vi "Acquisizione corse trigger.vi"() -> ()   [LabVIEW 2017]
uses:
  <vilib>/DAQmx/read.llb/DAQmx Read (Analog 1D Wfm NChan NSamp).vi
  <vilib>/Waveform/WDTOps.llb/WDT Index Channel DBL.vi
  <vilib>/Waveform/WDTOps.llb/WDT Append Waveforms DBL.vi
  <resource>/objmgr/daqmx.rc
  <vilib>/DAQmx/configure/timing.llb/DAQmx Timing (Sample Clock).vi
  <vilib>/DAQmx/configure/trigger.llb/DAQmx Start Trigger (Analog Edge).vi
  <vilib>/DAQmx/configure/trigger.llb/DAQmx Reference Trigger (Analog Edge).vi
panel:
  in  "source":string
  in  "rate":dbl=1000.0 format="%0.2f"
  in  "sample mode":i32(ring)=10178 items=["Finite Samples"=10178, "Continuous Samples"=10123, "Hardware Timed Single Point"=12522]
  in  "samples per channel":i32=1000
  in  "Save":bool
  out "error out":errorcluster
  in  "error in (no error)":errorcluster
  in  "valore di controllo 2":dbl=4.0
  in  "index 2":i32=2
  in  "valore di controllo":dbl=4.0
  in  "index":i32=2
  out "Photocell B":waveform(dbl)(graph)
  out "Photocell A":waveform(dbl)(graph)
  in  "Massa":string="_"
  out "photocell A":bool
  out "photocell B":bool
  in  "directory":path
  out "Load_Cell":waveform(dbl)(graph)
  in  "On/off":bool
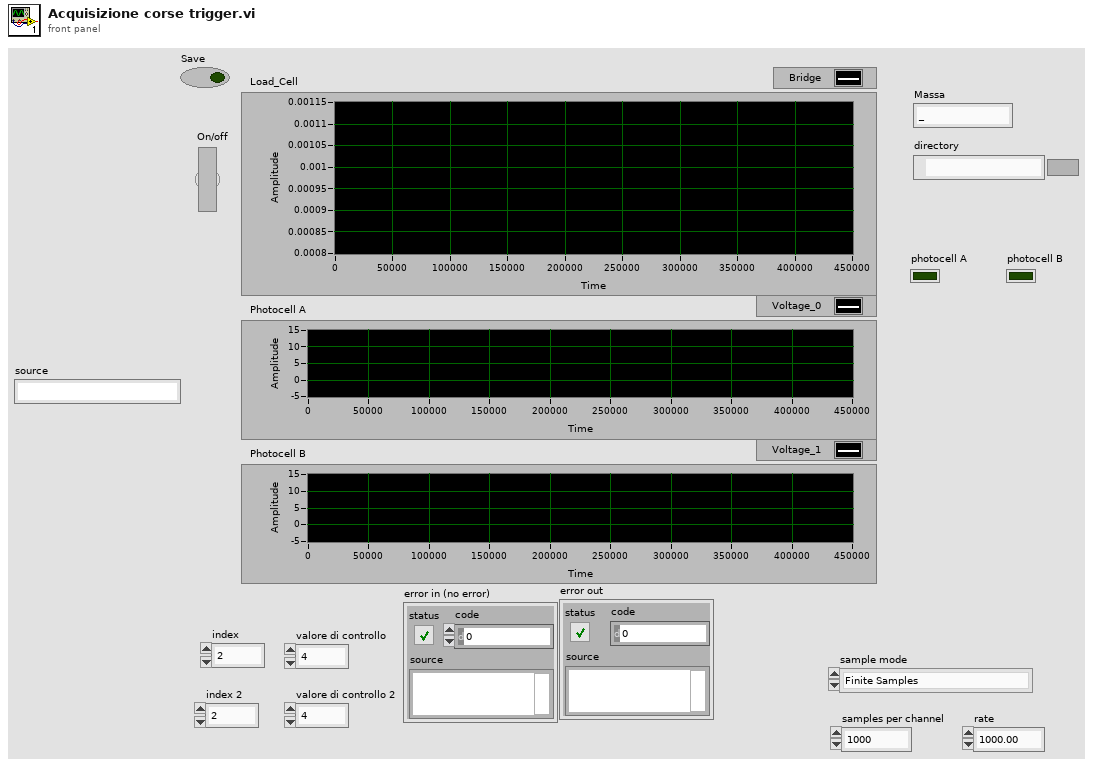
[diagram p1: front panel]
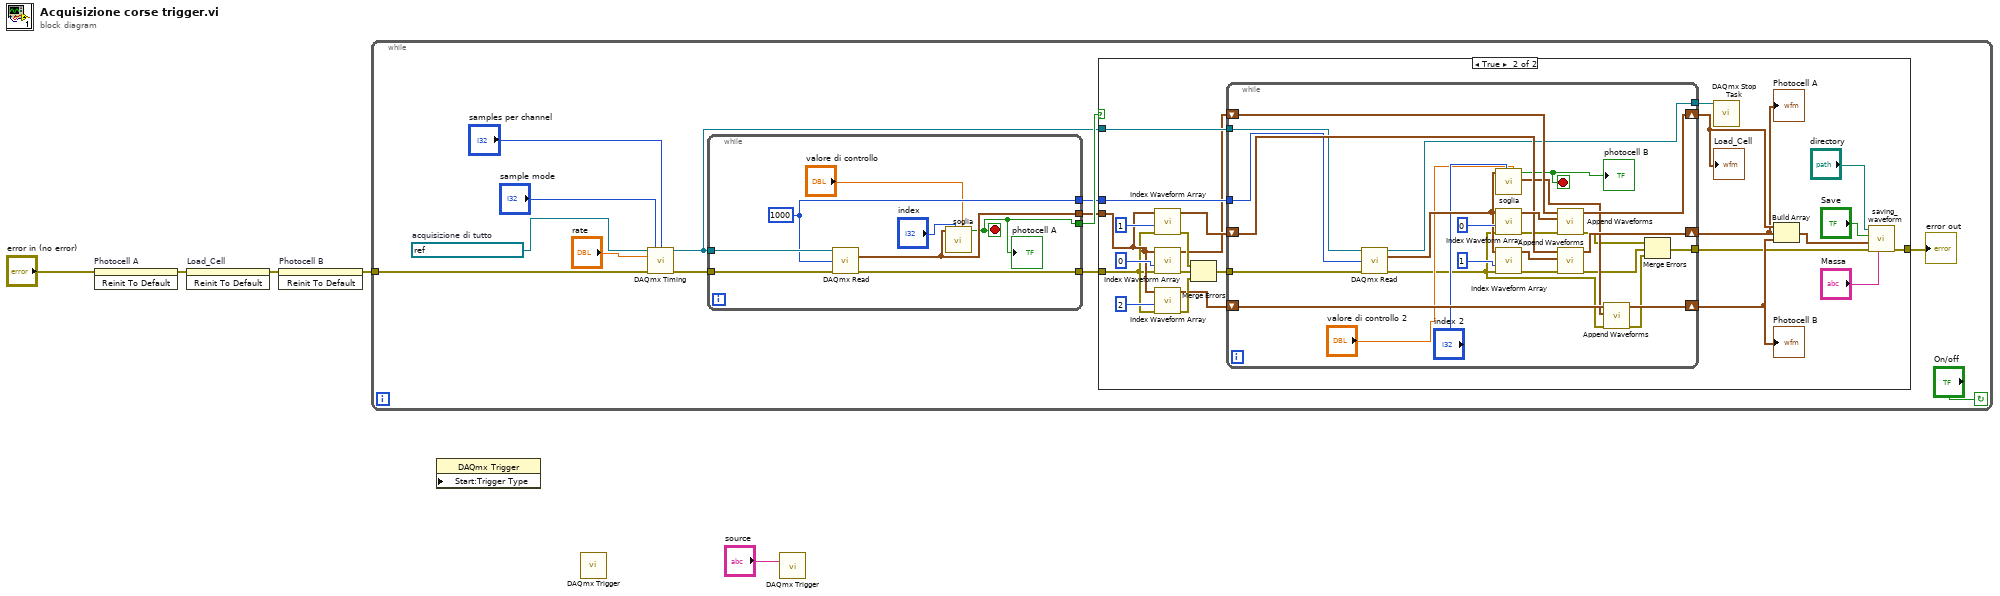
[diagram p0: block diagram]
diagram:
  n1 = invoke on="Photocell A" class="WFGraph (strict)" method="Reinit To Default"(error in="error in (no error)") -> (error out=w4:errorcluster)  [unwired: 2 in, 2 out]
  n2 = invoke on="Load_Cell" class="WFGraph (strict)" method="Reinit To Default"(error in=w4) -> (error out=w3:errorcluster)  [unwired: 2 in, 2 out]
  n3 = invoke on="Photocell B" class="WFGraph (strict)" method="Reinit To Default"(error in=w3) -> (error out=w2:errorcluster)  [unwired: 2 in, 2 out]
  n4 = while {
    tunnel: w2 -> [w6]
    stop <- "On/off" continue-if-true
    w7 = refnum<k21> "NastroTrasportatore"  # acquisizione di tutto
    n5 = call-poly <vilib>:"DAQmx Timing.vi"("task/channels in"=w7, "sample mode"="sample mode", "samples per channel"="samples per channel", "rate"="rate", "error in"=w6) -> ("task out"=w12:refnum<k21>, "error out"=w11:errorcluster)  [unwired: 9 in]
    n6 = while {
      tunnel: [w23] -> w17
      tunnel: [w26] -> w16
      tunnel: w12 -> [w25]
      tunnel: [w24] -> w15
      tunnel: w11 -> [w20]
      tunnel: [w19] -> w14
      stop <- w23 stop-if-true
      w24 = 1000 ("number of samples per channel")
      n7 = call-poly <vilib>:"DAQmx Read.vi"("task/channels in"=w25, "number of samples per channel"=w24, "error in"=w20) -> ("data"=w26:waveform(dbl)[], "error out"=w19:errorcluster)  [unwired: 10 in, 1 out]
      n8 = call "soglia.vi"("valore di controllo"="valore di controllo", "index"="index", "waveform_in"=w26) -> ("Boolean"=w23:bool)  [unwired: 7 in, 1 out]
      "photocell A" <- w23
    }
    n9 = case shown="True" w17 {
      tunnel: w16 -> [_ w48]
      tunnel: w12 -> [_ w47]
      tunnel: w15 -> [_ w46]
      tunnel: w14 -> [w27 w38]
      tunnel: [w27 w31] -> w13
      frame False {
      }
      frame True {
        n10 = call-poly <vilib>:"Index Waveform Array.vi"("error in (no error)"=w38, "index"=1, "waveform array"=w48) -> ("error out"=w37:errorcluster, "waveform"=w30:waveform(dbl))  [unwired: 7 in]
        n11 = call-poly <vilib>:"Index Waveform Array.vi"("error in (no error)"=w38, "index"=0, "waveform array"=w48) -> ("error out"=w36:errorcluster, "waveform"=w29:waveform(dbl))  [unwired: 7 in]
        n12 = call-poly <vilib>:"Index Waveform Array.vi"("error in (no error)"=w38, "index"=2, "waveform array"=w48) -> ("error out"=w35:errorcluster, "waveform"=w28:waveform(dbl))  [unwired: 7 in]
        n13 = Merge Errors(w37, w36, w35) -> (w34:errorcluster)
        n14 = while {
          shift-right: [w73] -> w44
          shift-left: w29 -> [w74]
          shift-right: [w70] -> w43
          shift-left: w30 -> [w72]
          shift-right: [w68] -> w41
          shift-left: w28 -> [w69]
          tunnel: w47 -> [w67]
          tunnel: w46 -> [w66]
          tunnel: [w65] -> w45
          tunnel: w34 -> [w59]
          tunnel: [w52] -> w32
          stop <- w63 stop-if-true
          n15 = call-poly <vilib>:"DAQmx Read.vi"("task/channels in"=w67, "number of samples per channel"=w66, "error in"=w59) -> ("task out"=w65:refnum<k21>, "data"=w64:waveform(dbl)[], "error out"=w56:errorcluster)  [unwired: 10 in]
          n16 = call "soglia.vi"("valore di controllo"="valore di controllo 2", "index"="index 2", "waveform_in"=w64) -> ("waveform_out_single"=w62:waveform(dbl), "Boolean"=w63:bool)  [unwired: 7 in]
          "photocell B" <- w63
          n17 = call-poly <vilib>:"Index Waveform Array.vi"("error in (no error)"=w56, "index"=0, "waveform array"=w64) -> ("error out"=w57:errorcluster, "waveform"=w75:waveform(dbl))  [unwired: 7 in]
          n18 = call-poly <vilib>:"Index Waveform Array.vi"("error in (no error)"=w56, "index"=1, "waveform array"=w64) -> ("error out"=w58:errorcluster, "waveform"=w71:waveform(dbl))  [unwired: 7 in]
          n19 = call-poly <vilib>:"Append Waveforms.vi"("error in (no error)"=w57, "waveform B"=w75, "waveform A"=w74) -> ("error out"=w55:errorcluster, "waveform out"=w73:waveform(dbl))  [unwired: 7 in]
          n20 = call-poly <vilib>:"Append Waveforms.vi"("error in (no error)"=w58, "waveform B"=w71, "waveform A"=w72) -> ("error out"=w54:errorcluster, "waveform out"=w70:waveform(dbl))  [unwired: 7 in]
          n21 = call-poly <vilib>:"Append Waveforms.vi"("error in (no error)"=w56, "waveform B"=w62, "waveform A"=w69) -> ("error out"=w53:errorcluster, "waveform out"=w68:waveform(dbl))  [unwired: 7 in]
          n22 = Merge Errors(w55, w54, w53) -> (w52:errorcluster)
        }
        "Load_Cell" <- w44
        "Photocell A" <- w43
        "Photocell B" <- w41
        n23 = call <vilib>:"DAQmx Stop Task.vi"("task/channels in"=w45) -> ()  [unwired: 13 in, 2 out]
        n24 = Build Array(w44, w43, w41) -> (w42:waveform(dbl)[])
        n25 = call "saving_waveform.vi"("Massa"="Massa", "error in (no error)"=w32, "Array"=w42, "Save"="Save", "directory"="directory") -> ("error out"=w31:errorcluster)  [unwired: 6 in]
      }
    }
    "error out" <- w13
  }
  n26 = property class="DAQmx Trigger" props=["Start:Trigger Type"]() -> ()  [unwired: 3 in, 2 out]
  n27 = call-poly <vilib>:"DAQmx Trigger.vi"() -> ()  [unwired: 14 in, 2 out]
  n28 = call-poly <vilib>:"DAQmx Trigger.vi"("source"="source") -> ()  [unwired: 13 in, 2 out]
